vi "OLD Laser Control.vi"() -> ()   [LabVIEW 2012]
uses:
  <vilib>/DAQmx/write.llb/DAQmx Write (Analog DBL 1Chan 1Samp).vi
  <vilib>/Instr/_visa.llb/VISA Configure Serial Port (Instr).vi
  <vilib>/DAQmx/create/channels.llb/DAQmx Create Channel (AO-Voltage-Basic).vi
  <vilib>/DAQmx/miscellaneous.llb/DAQmx Fill In Error Info.vi
panel:
  out "V out":dbl
  in  "488 set":dbl min=0.0 max=1.0 step=0.1
  in  "488 power":dbl(slide) scale=0.0..1.0 scale format="%#_4g"
  out "488 SN":string
  in  "stop":bool
  in  "488":bool
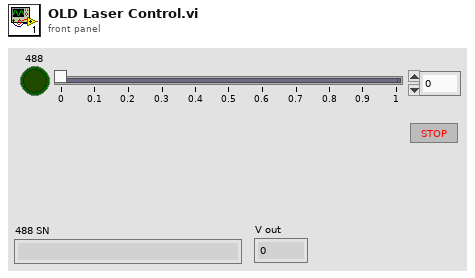
[diagram p1: front panel]
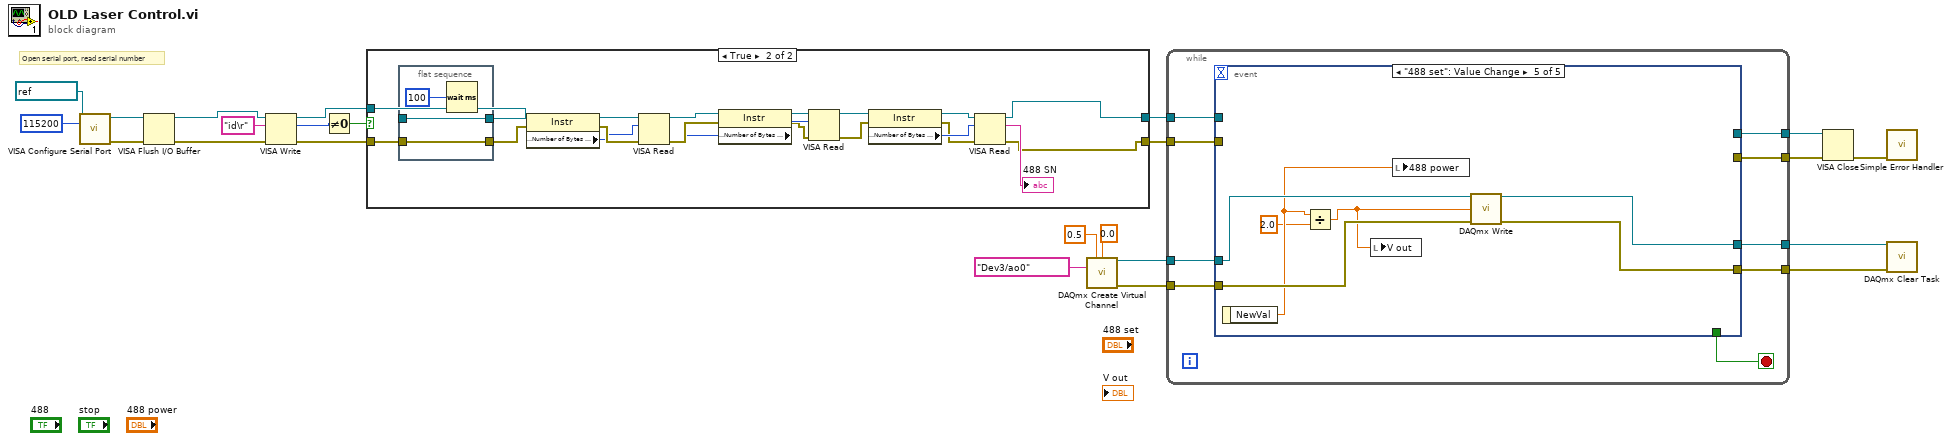
[diagram p0: block diagram]
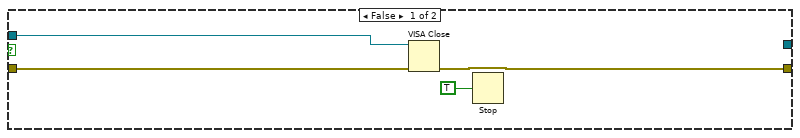
[diagram p2: hidden frame]
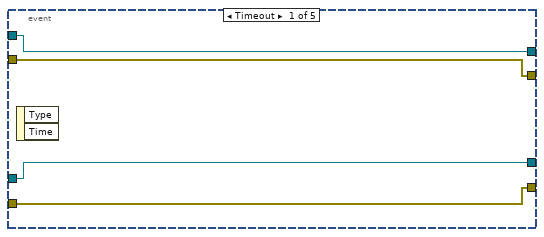
[diagram p3: hidden frame]
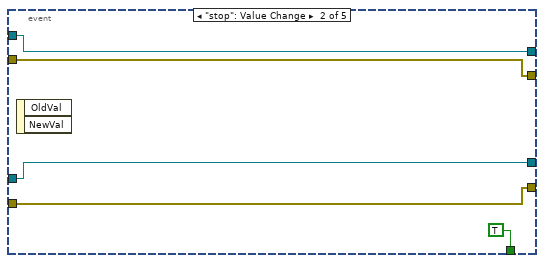
[diagram p4: hidden frame]
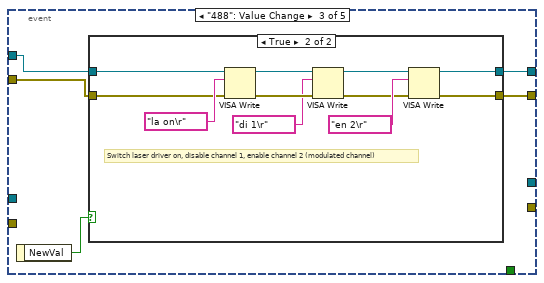
[diagram p5: hidden frame]
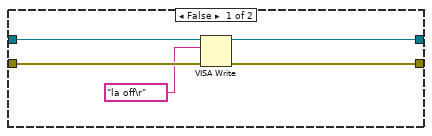
[diagram p6: hidden frame]
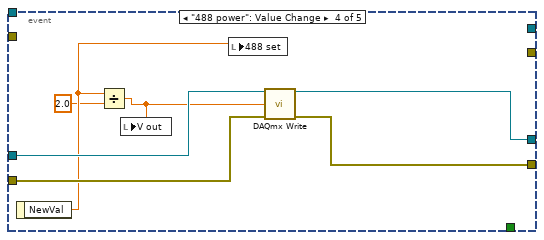
[diagram p7: hidden frame]
diagram:
  # "Open serial port, read serial number"
  n1 = call-poly "VISA Configure Serial Port"("VISA resource name"=refnum<visa-resource-name> "COM1", "baud rate (9600)"=u32 115200) -> ("VISA resource name out"=w9:refnum<visa-resource-name>, "error out"=w8:errorcluster)  [unwired: 12 in]
  n2 = VISA Flush I/O Buffer(VISA resource name=w9, error in (no error)=w8) -> (VISA resource name out=w11:refnum<visa-resource-name>, error out=w10:errorcluster)  [unwired: 1 in]
  n3 = VISA Write(VISA resource name=w11, write buffer="id\r", error in (no error)=w10) -> (VISA resource name out=w15:refnum<visa-resource-name>, return count=w17:u32, error out=w14:errorcluster)
  n4 = Not Equal To 0?(x=w17) -> (x != 0?=w16:bool)
  n5 = case shown="True" w16 {
    tunnel: w15 -> [w24 w47]
    tunnel: w14 -> [w27 w46]
    tunnel: [_ w31] -> w23
    tunnel: [w25 w30] -> w22
    frame False {
      n6 = VISA Close(VISA resource name=w24, error in (no error)=w27) -> (error out=w25:errorcluster)
      n7 = Stop(stop? (T)=TRUE) -> ()
    }
    frame True {
      n8 = flat-sequence {
        tunnel: [w49] -> w45
        tunnel: w47 -> [w49]
        tunnel: [w48] -> w44
        tunnel: w46 -> [w48]
        frame #0 {
          n9 = Wait (ms)(milliseconds to wait=u32 100) -> ()  [unwired: 1 out]
        }
      }
      n10 = property class="Instr"(reference=w45, error in=w44) -> (reference out=w43:refnum<visa-resource-name>, error out=w42:errorcluster, "Serial Settings:Number of Bytes at Serial Port"=w41:u32)
      n11 = VISA Read(VISA resource name=w43, byte count=w41, error in (no error)=w42) -> (VISA resource name out=w40:refnum<visa-resource-name>, error out=w39:errorcluster)  [unwired: 2 out]
      n12 = property class="Instr"(reference=w40, error in=w39) -> (reference out=w38:refnum<visa-resource-name>, error out=w36:errorcluster, "Serial Settings:Number of Bytes at Serial Port"=w37:u32)
      n13 = VISA Read(VISA resource name=w38, byte count=w37, error in (no error)=w36) -> (VISA resource name out=w35:refnum<visa-resource-name>, error out=w34:errorcluster)  [unwired: 2 out]
      n14 = property class="Instr"(reference=w35, error in=w34) -> (reference out=w29:refnum<visa-resource-name>, error out=w28:errorcluster, "Serial Settings:Number of Bytes at Serial Port"=w33:u32)
      n15 = VISA Read(VISA resource name=w29, byte count=w33, error in (no error)=w28) -> (VISA resource name out=w31:refnum<visa-resource-name>, read buffer=→"488 SN":string, error out=w30:errorcluster)  [unwired: 1 out]
    }
  }
  n16 = call-poly <vilib>:"DAQmx Create Virtual Channel.vi"("maximum value"=0.5, "minimum value"=0.0, "physical channels"=tag "Dev3/ao0") -> ("task out"=w4:refnum<k21>, "error out"=w3:errorcluster)  [unwired: 11 in]
  n17 = while {
    tunnel: w23 -> [w58]
    tunnel: w22 -> [w57]
    tunnel: [w56] -> w21
    tunnel: [w55] -> w20
    tunnel: w4 -> [w54]
    tunnel: w3 -> [w53]
    tunnel: [w52] -> w2
    tunnel: [w51] -> w1
    stop <- w59 stop-if-true
    n18 = event shown="[4] \"488 set\": Value Change" {
      selector: _ -> [_ _ _ _ _]
      dyn-events: _ -> [_ _ _ _ _]
      timeout: _ -> [_ _ _ _ _]
      tunnel: [_ TRUE _ _ _] -> w59
      tunnel: w58 -> [w63 w67 w72 _ _]
      tunnel: w57 -> [w62 w66 w71 _ _]
      tunnel: [w63 w67 w70 _ _] -> w56
      tunnel: [w62 w66 w69 _ _] -> w55
      tunnel: w54 -> [w61 w65 _ w96 w103]
      tunnel: w53 -> [w60 w64 _ w95 w102]
      tunnel: [w61 w65 _ w94 w101] -> w52
      tunnel: [w60 w64 _ w93 w100] -> w51
      event Timeout {
        n19 = event-data() -> ()  [unwired: 1 in, 2 out]
      }
      event "stop": Value Change {
        n20 = event-data() -> ()  [unwired: 1 in, 2 out]
      }
      event "488": Value Change {
        n21 = event-data() -> ("NewVal"=w73:bool)  [unwired: 1 in]
        n22 = case shown="True" w73 {
          tunnel: w72 -> [w78 w88]
          tunnel: w71 -> [w77 w87]
          tunnel: [w76 w80] -> w70
          tunnel: [w75 w79] -> w69
          frame False {
            n23 = VISA Write(VISA resource name=w78, write buffer="la off\r", error in (no error)=w77) -> (VISA resource name out=w76:refnum<visa-resource-name>, error out=w75:errorcluster)  [unwired: 1 out]
          }
          frame True {
            # "Switch laser driver on, disable channel 1, enable channel 2 (modulated channel)"
            n24 = VISA Write(VISA resource name=w88, write buffer="la on\r", error in (no error)=w87) -> (VISA resource name out=w86:refnum<visa-resource-name>, error out=w85:errorcluster)  [unwired: 1 out]
            n25 = VISA Write(VISA resource name=w86, write buffer="di 1\r", error in (no error)=w85) -> (VISA resource name out=w82:refnum<visa-resource-name>, error out=w81:errorcluster)  [unwired: 1 out]
            n26 = VISA Write(VISA resource name=w82, write buffer="en 2\r", error in (no error)=w81) -> (VISA resource name out=w80:refnum<visa-resource-name>, error out=w79:errorcluster)  [unwired: 1 out]
          }
        }
      }
      event "488 power": Value Change {
        n27 = event-data() -> ("NewVal"=w92:dbl)  [unwired: 1 in]
        n28 = Divide(x=w92, y=2.0) -> (x/y=w90:dbl)
        n29 = local write "V out"(w90) -> ()
        n30 = local write "488 set"(w92) -> ()
        n31 = call-poly <vilib>:"DAQmx Write.vi"("task/channels in"=w96, "data"=w90, "error in"=w95) -> ("task out"=w94:refnum<k21>, "error out"=w93:errorcluster)  [unwired: 10 in, 1 out]
      }
      event "488 set": Value Change {
        n32 = event-data() -> ("NewVal"=w99:dbl)  [unwired: 1 in]
        n33 = Divide(x=w99, y=2.0) -> (x/y=w98:dbl)
        n34 = local write "V out"(w98) -> ()
        n35 = local write "488 power"(w99) -> ()
        n36 = call-poly <vilib>:"DAQmx Write.vi"("task/channels in"=w103, "data"=w98, "error in"=w102) -> ("task out"=w101:refnum<k21>, "error out"=w100:errorcluster)  [unwired: 10 in, 1 out]
      }
    }
  }
  n37 = VISA Close(VISA resource name=w21, error in (no error)=w20) -> (error out=w12:errorcluster)
  n38 = call <vilib>:"Simple Error Handler.vi"("error in (no error)"=w12) -> ()  [unwired: 1 in, 8 out]
  n39 = call <vilib>:"DAQmx Clear Task.vi"("task in"=w2, "error in"=w1) -> ()  [unwired: 13 in, 1 out]
